vi "StreamReader.vi"(8 "error in (no error)":errorcluster, 10 "Stream":string, 11 "UserData":variant) -> (0 "error out":errorcluster)   [LabVIEW 2014]
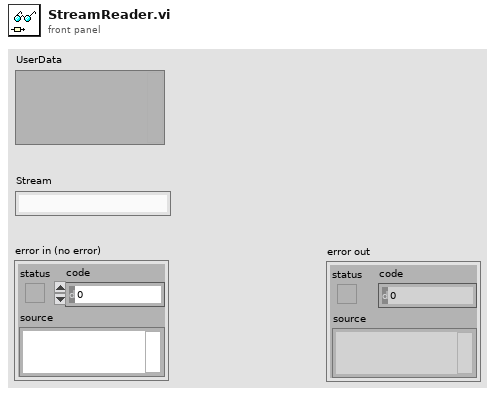
[diagram p1: front panel]
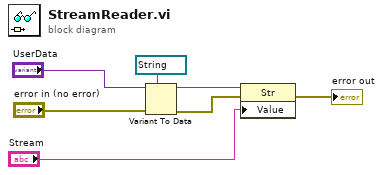
[diagram p0: block diagram]
diagram:
  n1 = Variant To Data(error in="error in (no error)", type=refnum<vi> refnum ("Stream"), Variant="UserData") -> (data=w4:refnum<vi>, error out=w3:errorcluster)
  n2 = property class="Str"(reference=w4, error in=w3, "Value"="Stream") -> (error out=→"error out":errorcluster)  [unwired: 1 out]
